vi "Prober_InitialiseUI.vi"(8 "error in (no error)":errorcluster, 11 "TeslaVeloxProbeStation in":refnum<class "TeslaVeloxProbeStation.lvclass">) -> (0 "error out":errorcluster, 2 "Probestation Configuration":variant, 3 "TeslaVeloxProbeStation out":refnum<class "TeslaVeloxProbeStation.lvclass">)   [LabVIEW 2018, in "TeslaVeloxProbeStation.lvclass"]
uses:
  TeslaVeloxProbeStation.lvclass
  TeslaVelox_GlobalConfig.vi
panel:
  out "Connected device (ResourceName)":string
  in  "Stop Button":bool
  in  "Condition 3":bool=TRUE
  in  "Condition 2":bool=TRUE
  in  "Condition 1":bool=TRUE
  # "Starting Probe Station Control Interface"
  # "This step will register the labview application to the VELOX software. If the labview was not exitted properly with (proper close of communitation), it will fail and disconnect properly. Next time it should work."
  # "Before continuing, please confirm the following:"
  # "1. Velox is running on the probestation PC"
  # "2. Sensor is contacted by the flying probe"
  # "Probe needle is properly aligned and at correct height"
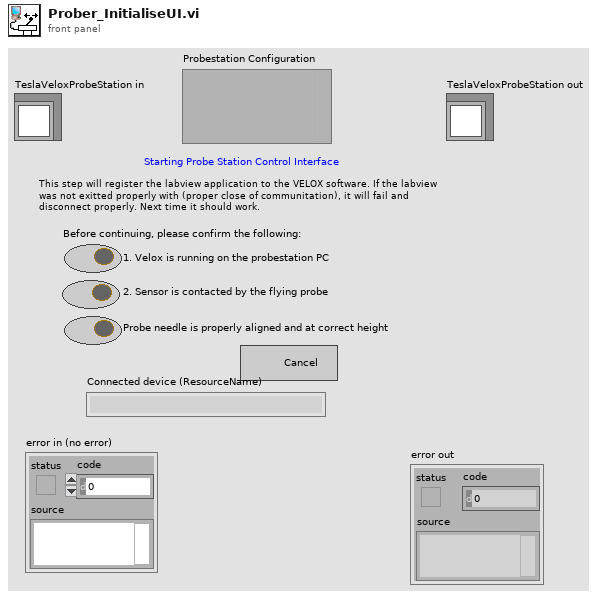
[diagram p1: front panel]
types:
  T1 = cluster{"IP address":string, "Separation gap[um]":dbl, "Port Number":i32, "Use Overdrive?":bool, "Touchdown method":enum16{"no feedback"}, "Coordinate system":enum16{"Cartesian", "X as index"}}
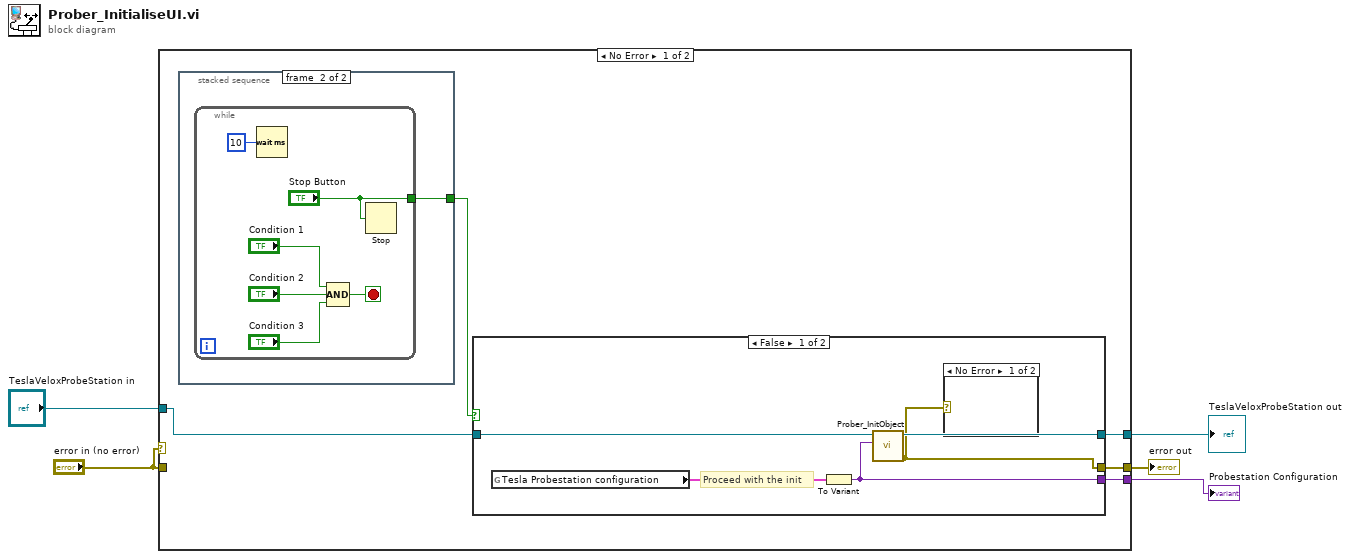
[diagram p0: block diagram]
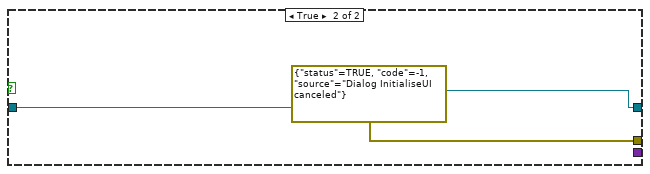
[diagram p3: hidden frame]
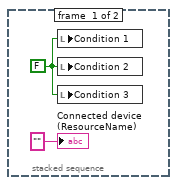
[diagram p4: hidden frame]
diagram:
  n1 = case shown="No Error" "error in (no error)" {
    tunnel: "error in (no error)" -> [_ w27]
    tunnel: "TeslaVeloxProbeStation in" -> [w7 w28]
    tunnel: [w8 _] -> w3
    tunnel: [w9 w27] -> w2
    tunnel: [w6 w28] -> w1
    frame No Error {
      n2 = stacked-sequence {
        tunnel: [_ w20] -> w10
        frame #0 {
          w18 = FALSE ("Condition 1")
          n3 = local write "Condition 1"(w18) -> ()
          n4 = local write "Condition 2"(w18) -> ()
          n5 = local write "Condition 3"(w18) -> ()
          "Connected device (ResourceName)" <- "" ("Connected device (ResourceName)")
        }
        frame #1 {
          n6 = while {
            tunnel: ["Stop Button"] -> w20
            stop <- w21 stop-if-true
            n7 = Wait (ms)(milliseconds to wait=u32 10) -> ()  [unwired: 1 out]
            n8 = Compound Arithmetic op=AND("Condition 1", "Condition 2", "Condition 3") -> (w21:bool)
            n9 = Stop(stop? (T)="Stop Button") -> ()
          }
        }
      }
      n10 = case shown="False" w10 {
        tunnel: [w11 errorcluster {"status"=TRUE, "code"=-1, "source"="Dialog InitialiseUI canceled"} ("error out")] -> w9
        tunnel: [w15 _] -> w8
        tunnel: w7 -> [w14 w16]
        tunnel: [w13 w16] -> w6
        frame False {
          # "Proceed with the init"
          n11 = global read "TeslaVelox_GlobalConfig.vi" "Tesla Probestation configuration"() -> (w12:T1)
          n12 = To Variant(anything=w12) -> (Variant=w15:variant)
          n13 = call-dynamic "Prober_InitObject.vi"("Prober Configuration"=w15, "TeslaVeloxProbeStation in"=w14) -> ("error out"=w11:errorcluster, "TeslaVeloxProbeStation out"=w13:refnum<class "TeslaVeloxProbeStation.lvclass">)  [unwired: 8 in]
          n14 = case shown="No Error" w11 {
            frame No Error {
            }
            frame Error {
            }
          }
        }
        frame True {
          # "cancled"
        }
      }
    }
    frame Error {
    }
  }
  "error out" <- w2
  "TeslaVeloxProbeStation out" <- w1
  "Probestation Configuration" <- w3
